vi "Plot Vibration.vi"(8 "IntensityGraph in 2":refnum<vi>, 9 "External Data TD":T1, 10 "sampling rate":dbl=5120.0 format="%#_13g", 11 "IntensityGraph in":refnum<vi>) -> (2 "STFT Spectrogram 2":dbl[][](graph), 3 "STFT Spectrogram":dbl[][](graph))   [LabVIEW 2016]
uses:
  Vibration data TD.ctl
  <vilib>/gmath/NI_Gmath.lvlib
panel:
  in  "step size":i32=256
  in  "FFT size":i32=1024
  in  "window length":i32=512
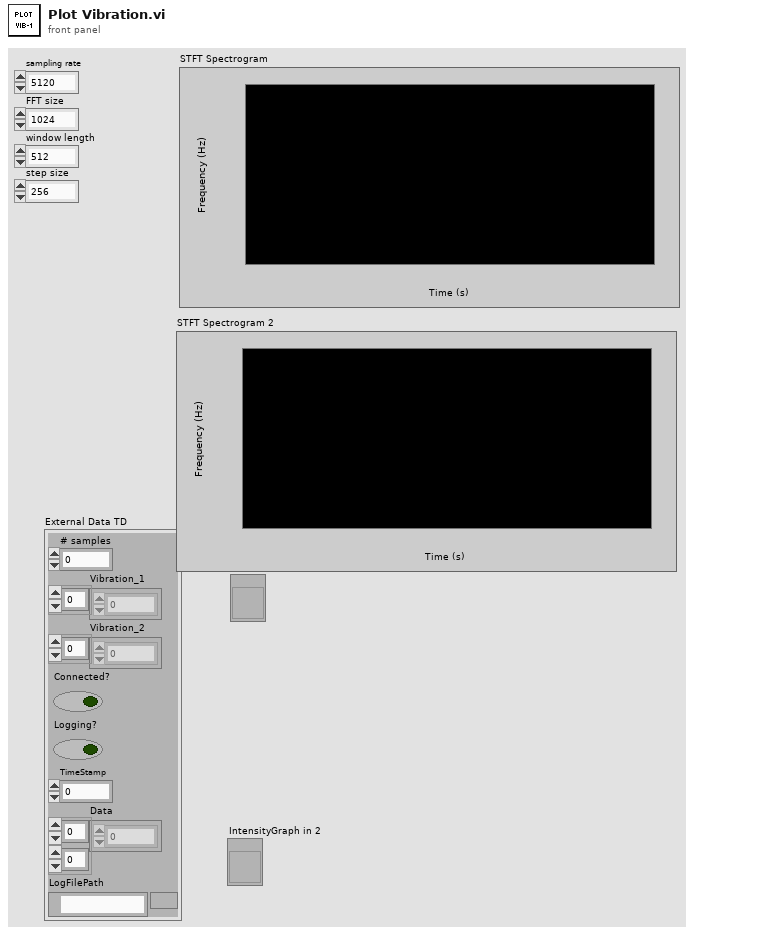
[diagram p1: front panel]
types:
  T1 = typedef "Vibration data TD.ctl" = cluster{"# samples":i32, "Vibration_1":dbl[], "Vibration_2":dbl[], "Connected?":bool, "Logging?":bool, "TimeStamp":dbl, "Data":dbl[][], "LogFilePath":path}
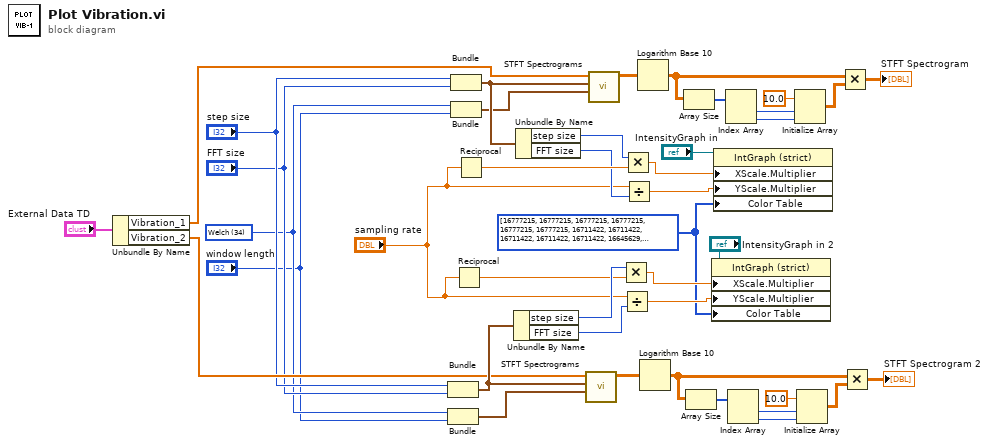
[diagram p0: block diagram]
diagram:
  w6 = u32[] [16777215, 16777215, 16777215, 16777215, 16777215, 16777215, 16711422, 16711422, 16711422, 16711422, 16711422, 16645629, 16645629, 16645629, 16645629, 16645629, 16645629, 16579836, 16579836, 16579836, 16579836, 16579836, 16514043, 16514043, 16514043, 16514043, 16514043, 16448250, 16448250, 16448250, 16448250, 16448250, 16316664, 16382457, 16382457, 16382457, 16382457, 16316664, 16316664, 16316664, 16316664, 16250871, 16250871, 16250871, 16250871, 16250871, 16185078, 16185078, 16185078, 16185078, 16119285, 16119285, 16119285, 16119285, 16119285, 16053492, 16053492, 16053492, 16053492, 15987699, 15987699, 15987699, 15987699, 15921906, 15987699, 15921906, 15921906, 15856113, 15856113, 15856113, 15856113, 15856113, 15790320, 15790320, 15790320, 15724527, 15724527, 15724527, 15724527, 15658734, 15658734, 15658734, 15658734, 15592941, 15592941, 15592941, 15592941, 15527148, 15527148, 15527148, 15461355, 15461355, 15461355, 15461355, 15395562, 15395562, 15395562, 15395562, 15329769, 15329769, 15329769, 15263976, 15263976, 15263976, 15198183, 15198183, 15198183, 15198183, 15132390, 15132390, 15132390, 15066597, 15066597, 15066597, 15000804, 15000804, 15000804, 14935011, 14935011, 14935011, 14869218, 14869218, 14869218, 14803425, 14803425, 14803425, 14737632, 14737632, 14671839, 14671839, 14671839, 14606046, 14606046, 14606046, 14540253, 14540253, 14540253, 14474460, 14474460, 14408667, 14408667, 14408667, 14342874, 14342874, 14277081, 14277081, 14277081, 14211288, 14211288, 14145495, 14145495, 14079702, 14079702, 14013909, 14013909, 14013909, 13948116, 13948116, 13882323, 13882323, 13816530, 13816530, 13750737, 13750737, 13684944, 13684944, 13619151, 13619151, 13553358, 13553358, 13487565, 13487565, 13421772, 13421772, 13355979, 13290186, 13290186, 13224393, 13224393, 13158600, 13092807, 13092807, 13027014, 13027014, 12961221, 12895428, 12895428, 12829635, 12763842, 12763842, 12698049, 12632256, 12566463, 12566463, 12500670, 12434877, 12434877, 12369084, 12303291, 12237498, 12171705, 12171705, 12105912, 12040119, 11974326, 11908533, 11842740, 11776947, 11711154, 11645361, 11579568, 11513775, 11447982, 11382189, 11316396, 11250603, 11184810, 11119017, 10987431, 10921638, 10855845, 10790052, 10658466, 10592673, 10461087, 10395294, 10329501, 10197915, 10066329, 10000536, 9868950, 9737364, 9605778, 9474192, 9342606, 9211020, 9079434, 8882055, 8750469, 8553090, 8421504, 8224125, 7960953, 7763574, 7500402, 7237230, 6974058, 6645093, 6316128, 5855577, 5395026, 4868682, 4210752, 3289650, 2105376, 0] ("256 log up")
  w2 = u32 34 items=["Rectangle"=0, "Hanning"=1, "Hamming"=2, "Blackman-Harris"=3, "Exact Blackman"=4, "Blackman"=5, "Flat Top"=6, "4 Term B-Harris "=7, "7 Term B-Harris"=8, "Low Sidelobe"=9, "Blackman Nuttall"=11, "Triangle"=30, "Bartlett-Hanning"=31, "Bohman"=32, "Parzen"=33, "Welch"=34, "Kaiser"=60, "Dolph-Chebyshev"=61, "Gaussian"=62] ("Type")
  n1 = Unbundle By Name("External Data TD") -> ("Vibration_1"=w23:dbl[], "Vibration_2"=w24:dbl[])
  n2 = Bundle("step size"="step size", "FFT size"="FFT size") -> (w25:cluster{"step size":i32, "FFT size":i32})  [unwired: 1 in]
  n3 = Bundle("Type"=w2, "window length"="window length") -> (w31:cluster{"Type":u32, "window length":i32})  [unwired: 1 in]
  n4 = Bundle("step size"="step size", "FFT size"="FFT size") -> (w41:cluster{"step size":i32, "FFT size":i32})  [unwired: 1 in]
  n5 = Bundle("Type"=w2, "window length"="window length") -> (w35:cluster{"Type":u32, "window length":i32})  [unwired: 1 in]
  n6 = Reciprocal(x="sampling rate") -> (1/x=w26:dbl)
  n7 = Reciprocal(x="sampling rate") -> (1/x=w40:dbl)
  n8 = Unbundle By Name(w25) -> ("step size"=w30:i32, "FFT size"=w29:i32)
  n9 = Unbundle By Name(w41) -> ("step size"=w36:i32, "FFT size"=w37:i32)
  n10 = call <vilib>:"STFT Spectrograms.vi"("window info"=w31, "time-freq sampling info"=w25, "X"=w24) -> ("STFT Spectrogram {X}"=w8:dbl[][])  [unwired: 3 in, 5 out]
  n11 = call <vilib>:"STFT Spectrograms.vi"("window info"=w35, "time-freq sampling info"=w41, "X"=w23) -> ("STFT Spectrogram {X}"=w16:dbl[][])  [unwired: 3 in, 5 out]
  n12 = Multiply(x=w30, y=w26) -> (x*y=w28:dbl)
  n13 = Divide(x="sampling rate", y=w29) -> (x/y=w27:dbl)
  n14 = Multiply(x=w36, y=w40) -> (x*y=w38:dbl)
  n15 = Divide(x="sampling rate", y=w37) -> (x/y=w39:dbl)
  n16 = Logarithm Base 10(1:w16) -> (0:w17:dbl[][])
  n17 = Logarithm Base 10(1:w8) -> (0:w14:dbl[][])
  n18 = Array Size(array=w17) -> (size(s)=w22:i32[])
  n19 = Array Size(array=w14) -> (size(s)=w9:i32[])
  n20 = property on="Property Node" class="IntGraph (strict)"(reference="IntensityGraph in 2", "XScale.Multiplier"=w28, "YScale.Multiplier"=w27, "Color Table"=w6) -> ()  [unwired: 1 in, 2 out]
  n21 = property on="Property Node" class="IntGraph (strict)"(reference="IntensityGraph in", "XScale.Multiplier"=w38, "YScale.Multiplier"=w39, "Color Table"=w6) -> ()  [unwired: 1 in, 2 out]
  n22 = Index Array(array=w22) -> (element #1=w21:i32, element #2=w20:i32)  [unwired: 2 in]
  n23 = Index Array(array=w9) -> (element #1=w10:i32, element #2=w11:i32)  [unwired: 2 in]
  n24 = Initialize Array(10.0, w21, w20) -> (w18:dbl[][])
  n25 = Initialize Array(10.0, w10, w11) -> (w13:dbl[][])
  n26 = Multiply(x=w17, y=w18) -> (x*y=→"STFT Spectrogram":dbl[][])
  n27 = Multiply(x=w14, y=w13) -> (x*y=→"STFT Spectrogram 2":dbl[][])
